vi "EnableDisable - Right Click.vi"(8 "error in (no error)":errorcluster, 11 "Node Ptr":u64 format="%.0x") -> (0 "error out":errorcluster)   [LabVIEW 2012, in "AIT 429 System Explorer.lvlib"]
uses:
  AIT 429 System Explorer.lvlib
  Shared/Controls and Global/Global.vi
  <vilib>/NI Veristand/Custom Device API/Custom Device API.lvlib
  Shared/ARINC 429 Shared.lvlib
panel:
  in  "Tag":string
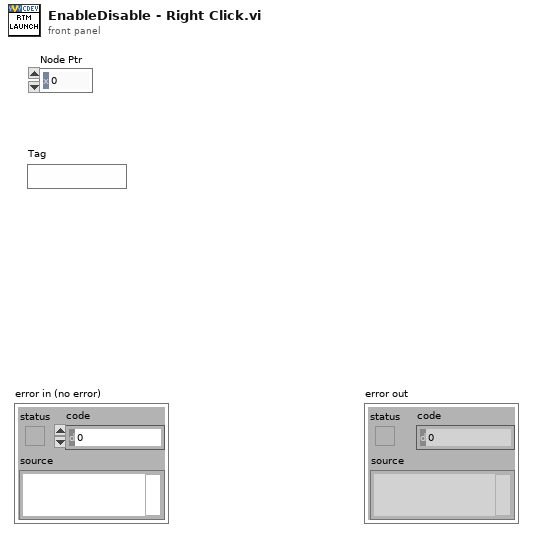
[diagram p1: front panel]
types:
  T1 = typedef "Custom Device API.lvlib/Custom Device Item Ref.ctl" = u64
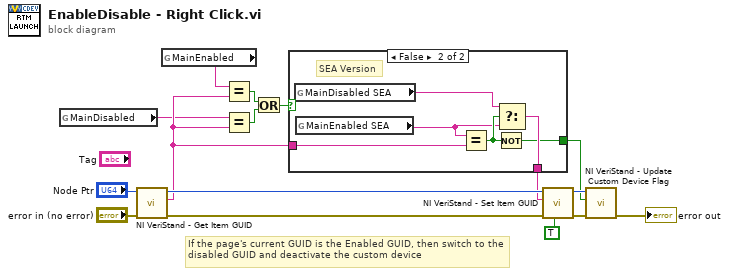
[diagram p0: block diagram]
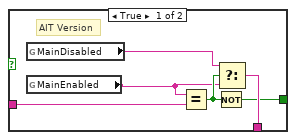
[diagram p2: hidden frame]
diagram:
  # "If the page's current GUID is the Enabled GUID, then switch to the disabled GUID and deactivate the custom device"
  n1 = global read "Global.vi" "MainDisabled"() -> (w4:string)
  n2 = call <vilib>:"NI VeriStand - Get Item GUID.vi"("error in (no error)"="error in (no error)", "Item Ref in"="Node Ptr") -> ("error out"=w15:errorcluster, "GUID"=w5:string, "Item Ref out"=w14:T1)  [unwired: 7 in]
  n3 = global read "Global.vi" "MainEnabled"() -> (w6:string)
  n4 = Equal?(x=w6, y=w5) -> (x = y?=w2:bool)
  n5 = Equal?(x=w4, y=w5) -> (x = y?=w1:bool)
  n6 = Or(x=w2, y=w1) -> (x .or. y?=w3:bool)
  n7 = case shown="False" w3 {
    tunnel: w5 -> [w22 w28]
    tunnel: [w21 w27] -> w13
    tunnel: [w19 w25] -> w10
    frame True {
      # "AIT Version"
      n8 = global read "Global.vi" "MainDisabled"() -> (w18:string)
      n9 = global read "Global.vi" "MainEnabled"() -> (w17:string)
      n10 = Equal?(x=w17, y=w22) -> (x = y?=w20:bool)
      n11 = Not(x=w20) -> (.not. x?=w19:bool)
      n12 = Select(t=w18, s=w20, f=w17) -> (s? t:f=w21:string)
    }
    frame False {
      # "SEA Version"
      n13 = global read "Global.vi" "MainDisabled SEA"() -> (w24:string)
      n14 = global read "Global.vi" "MainEnabled SEA"() -> (w23:string)
      n15 = Equal?(x=w23, y=w28) -> (x = y?=w26:bool)
      n16 = Not(x=w26) -> (.not. x?=w25:bool)
      n17 = Select(t=w24, s=w26, f=w23) -> (s? t:f=w27:string)
    }
  }
  n18 = call <vilib>:"NI VeriStand - Set Item GUID.vi"("Refresh System Explorer Tree? (F)"=TRUE, "error in (no error)"=w15, "GUID"=w13, "Item Ref in"=w14) -> ("error out"=w12:errorcluster, "Item Ref out"=w11:T1)  [unwired: 6 in]
  n19 = call <vilib>:"NI VeriStand - Update Custom Device Flag.vi"("error in (no error)"=w12, "Is Custom Device Active?"=w10, "Device Ref in"=w11) -> ("error out"=→"error out":errorcluster)  [unwired: 7 in, 1 out]
